vi "SmartMotor_Check InMotion State - single motor.vi"(8 "error in":errorcluster, 9 "ReadWait":u32=50, 10 "MotorSpecifier(None)":T1, 11 "VISA In":refnum<visa-resource-name>) -> (0 "error out":errorcluster, 2 "InMotion?":bool, 3 "VISA out":refnum<visa-resource-name>, 5 "cmd str out":string)   [LabVIEW 2020]
doc: "Developed by Kevin Thompson\nkevin@thompsonengineering.net\n\nCopyright 2018-2020\nThompson Engineering, LLC"
uses:
  TD SerialBusMotorSpecifier_enum.ctl
panel:
  in  "MotorSpecifier(None)":T1
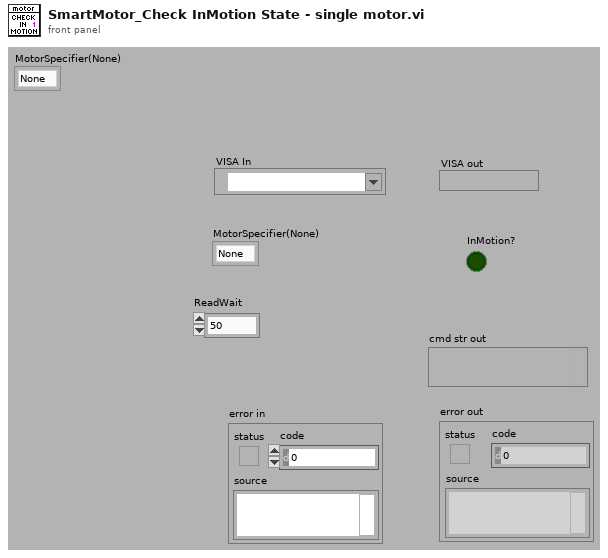
[diagram p1: front panel]
types:
  T1 = typedef "TD SerialBusMotorSpecifier_enum.ctl" = enum16{"None", "Global", "M1", "M2", "M3"}
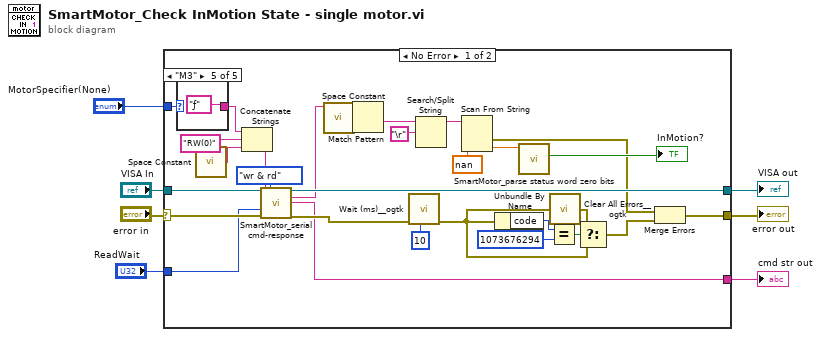
[diagram p0: block diagram]
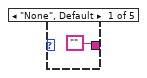
[diagram p2: hidden frame]
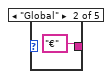
[diagram p3: hidden frame]
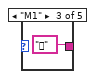
[diagram p4: hidden frame]
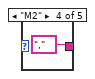
[diagram p5: hidden frame]
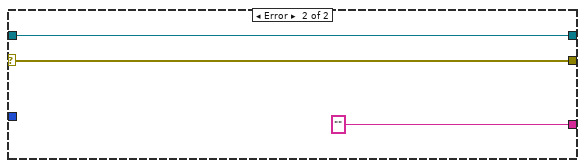
[diagram p6: hidden frame]
diagram:
  n1 = case shown="No Error" "error in" {
    selector: "error in" -> [w25 w43]
    tunnel: "VISA In" -> [w36 w44]
    tunnel: [w20 w44] -> w6
    tunnel: [w26 w43] -> w5
    tunnel: [w19 ""] -> w3
    tunnel: "MotorSpecifier(None)" -> [w16 _]
    tunnel: "ReadWait" -> [w8 _]
    frame No Error {
      n2 = case shown="\"M3\"" w16 {
        tunnel: ["" "€" "" "‚" "ƒ"] -> w17
        frame "None", Default {
        }
        frame "Global" {
        }
        frame "M1" {
        }
        frame "M2" {
        }
        frame "M3" {
        }
      }
      n3 = call <vilib>:"Space Constant.vi"() -> ("String"=w9:string)
      n4 = Concatenate Strings(w17, "RW(0)", w9) -> (w14:string)
      n5 = call "SmartMotor_serial cmd-response.vi"("VISA In"=w36, "mode"=enum16{"wr & rd", "write", "read"}."wr & rd", "cmd"=w14, "ReadWait"=w8, "error in"=w25) -> ("VISA out"=w20:refnum<visa-resource-name>, "str out"=w11:string, "cmd str out"=w19:string, "error out"=w22:errorcluster)  [unwired: 6 in, 1 out]
      n6 = call <vilib>:"Space Constant.vi"() -> ("String"=w12:string)
      n7 = Match Pattern(string=w11, regular expression=w12) -> (after substring=w10:string)  [unwired: 1 in, 3 out]
      n8 = call <userlib>:"Wait (ms)__ogtk.vi"("error in (no error)"=w22, "milliseconds to wait"=u32 10 ("wait (ms)")) -> ("error out"=w21:errorcluster)  [unwired: 8 in, 1 out]
      n9 = Search/Split String(string=w10, search string/char (-)="\r") -> (substring before match=w28:string)  [unwired: 3 out]
      n10 = Scan From String(input string=w28, default 1=nan ("measVal")) -> (error out=w18:errorcluster, output 1=w24:dbl)  [unwired: 3 in, 2 out]
      n11 = Unbundle By Name(w21) -> ("code"=w30:i32)
      n12 = call "SmartMotor_parse status word zero bits.vi"("SW0 in"=w24) -> ("InTrajMotion"=→"InMotion?":bool)  [unwired: 5 in, 5 out]
      n13 = Equal?(x=w30, y=1073676294 ("error code")) -> (x = y?=w32:bool)
      n14 = call <userlib>:"Clear All Errors__ogtk.vi"("Error In"=w21) -> ("Error Out"=w33:errorcluster)  [unwired: 3 in]
      n15 = Select(t=w33, s=w32, f=w21) -> (s? t:f=w27:errorcluster)
      n16 = Merge Errors(w18, w27) -> (w26:errorcluster)
    }
    frame Error {
    }
  }
  "VISA out" <- w6
  "error out" <- w5
  "cmd str out" <- w3
